vi "test Add and Remove UDP.vi"(8 "error in (no error)":errorcluster, 11 "TestCase in":refnum<class "Add and Remove Test.lvclass">) -> (0 "error out":errorcluster, 3 "TestCase out":refnum<class "Add and Remove Test.lvclass">)   [LabVIEW 2020, in "Add and Remove Test.lvclass"]
uses:
  Add and Remove Test.lvclass
  <vilib>/addons/_JKI Toolkits/VI Tester/TestCase.llb/TestCase.lvclass
  Scripting API/Data Sharing Framework Custom Device Scripting.lvlib
  Includes/DSF Core.lvlibp/Typedefs/DSF Timing Info.ctl
  Includes/DSF Core.lvlibp
  Includes/DSF Core.lvlibp/Typedefs/Core Plugin Configuration.ctl
  Includes/DSF Core.lvlibp/Classes/Configuration/Core/Plugin/Plugin Configuration.lvclass
  Includes/DSF Core.lvlibp/Typedefs/DSF Settings Info.ctl
  Includes/DSF Core.lvlibp/Typedefs/Core Thread Configuration.ctl
  Includes/DSF Core.lvlibp/Classes/Configuration/Core/Thread/Thread Configuration.lvclass
  Includes/DSF Core.lvlibp/Typedefs/DSF Direction.ctl
  Includes/DSF Core.lvlibp/Typedefs/DSF Timeout Behavior.ctl
  Includes/DSF Core.lvlibp/Typedefs/Core Group Configuration.ctl
  Includes/DSF Core.lvlibp/Classes/Configuration/Core/Group/Group Configuration.lvclass
  Includes/DSF Core.lvlibp/Typedefs/Core Transfer Configuration.ctl
  Includes/DSF Core.lvlibp/Classes/Configuration/Core/Transfer/Transfer Configuration.lvclass
  Includes/DSF Core.lvlibp/Typedefs/DSF Data Type.ctl
  Includes/DSF Core.lvlibp/Typedefs/Core Channel Configuration.ctl
  Includes/DSF Core.lvlibp/Classes/Configuration/Core/Channel/Channel Configuration.lvclass
  Includes/DSF Core.lvlibp/Typedefs/DSF Engine Channel Configuration.ctl
  Includes/DSF Core.lvlibp/Typedefs/DSF Engine Transfer Configuration.ctl
  Includes/DSF Core.lvlibp/Typedefs/DSF Engine Transfer Group Configuration.ctl
  Includes/DSF Core.lvlibp/Typedefs/DSF Engine Plugin Thread Configuration.ctl
  Includes/DSF Core.lvlibp/Typedefs/DSF Engine Plugin Configuration.ctl
  Includes/DSF Core.lvlibp/Typedefs/DSF Engine Framework Configuration.ctl
  <vilib>/NI/VeriStand Custom Device Testing Tools/VeriStandTestUtilities/VeriStandTestUtilities.lvlib
  Includes/DSF Core.lvlibp/Classes/Configuration Session/Configuration Session.lvclass
  <vilib>/NI VeriStand/Custom Device API/Custom Device Item Ref.ctl
  <vilib>/NI VeriStand/Custom Device API/Custom Device API.lvlib
  C:/Program Files (x86)/National Instruments/LabVIEW 2020/vi.lib/addons/_JKI Toolkits/VI Tester/TestCase.llb/TestCase.lvclass
  C:/Users/nitest/Desktop/Git/niveristand-data-sharing-framework-custom-device/Source/Custom Device/Tests/Unit/Add and Remove/Add and Remove Test.lvclass
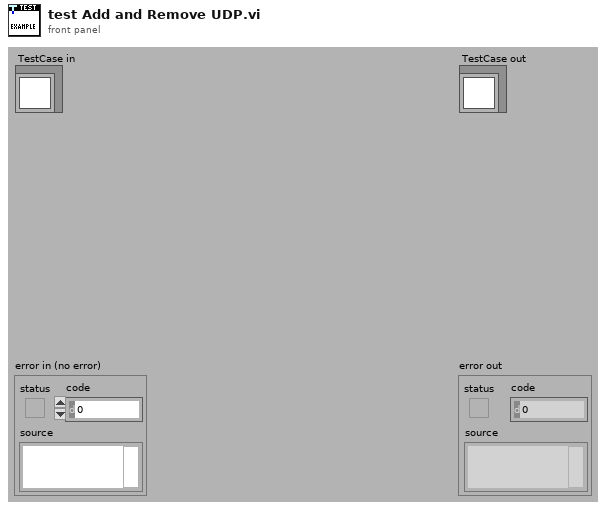
[diagram p1: front panel]
types:
  T1 = typedef "DSF Core.lvlibp/DSF Engine Framework Configuration.ctl" = cluster{"plugins":T2[]}
  T2 = typedef "DSF Core.lvlibp/DSF Engine Plugin Configuration.ctl" = cluster{"core":T3, "component settings":T5[], "threads":T6[]}
  T3 = typedef "DSF Core.lvlibp/Plugin Configuration.lvclass/Core Plugin Configuration.ctl" = cluster{"name":string, "components":string[], "cycle timing":T4}
  T4 = typedef "DSF Core.lvlibp/DSF Timing Info.ctl" = cluster{"priority":u64, "decimation":u64, "offset":u64}
  T5 = typedef "DSF Core.lvlibp/DSF Settings Info.ctl" = cluster{"component":string, "values":cluster{"key":string, "value":string}[]}
  T6 = typedef "DSF Core.lvlibp/DSF Engine Plugin Thread Configuration.ctl" = cluster{"core":T7, "component settings":T5[], "transfer groups":T8[]}
  T7 = typedef "DSF Core.lvlibp/Thread Configuration.lvclass/Core Thread Configuration.ctl" = cluster{"processor":i32, "priority offset":i16}
  T8 = typedef "DSF Core.lvlibp/DSF Engine Transfer Group Configuration.ctl" = cluster{"core":T9, "component settings":T5[], "transfers":T12[]}
  T9 = typedef "DSF Core.lvlibp/Group Configuration.lvclass/Core Group Configuration.ctl" = cluster{"name":string, "direction":T10, "cycle timing":T4, "timeout behavior":T11, "enable conversion":bool}
  T10 = typedef "DSF Core.lvlibp/DSF Direction.ctl" = enum8{"Tx", "Rx"}
  T11 = typedef "DSF Core.lvlibp/DSF Timeout Behavior.ctl" = enum8{"Increment Late Count", "Throw Error"}
  T12 = typedef "DSF Core.lvlibp/DSF Engine Transfer Configuration.ctl" = cluster{"core":T13, "component settings":T5[], "channels":T14[]}
  T13 = typedef "DSF Core.lvlibp/Transfer Configuration.lvclass/Core Transfer Configuration.ctl" = cluster{"name":string}
  T14 = typedef "DSF Core.lvlibp/DSF Engine Channel Configuration.ctl" = cluster{"core":T15, "component settings":T5[]}
  T15 = typedef "DSF Core.lvlibp/Channel Configuration.lvclass/Core Channel Configuration.ctl" = cluster{"name":string, "units":string, "engine data type":T16, "string data type":T16, "string offset":u64}
  T16 = typedef "DSF Core.lvlibp/DSF Data Type.ctl" = enum8{"Bool", "SGL", "DBL", "I8", "I16", "I32", "I64", "U8", "U16", "U32", "U64"}
  T17 = typedef "Custom Device API.lvlib/Custom Device Item Ref.ctl" = u64
  T18 = typedef "DSF Core.lvlibp/DSF Version Info.ctl" = cluster{"major":u32, "minor":u32, "fix":u32, "build":string}
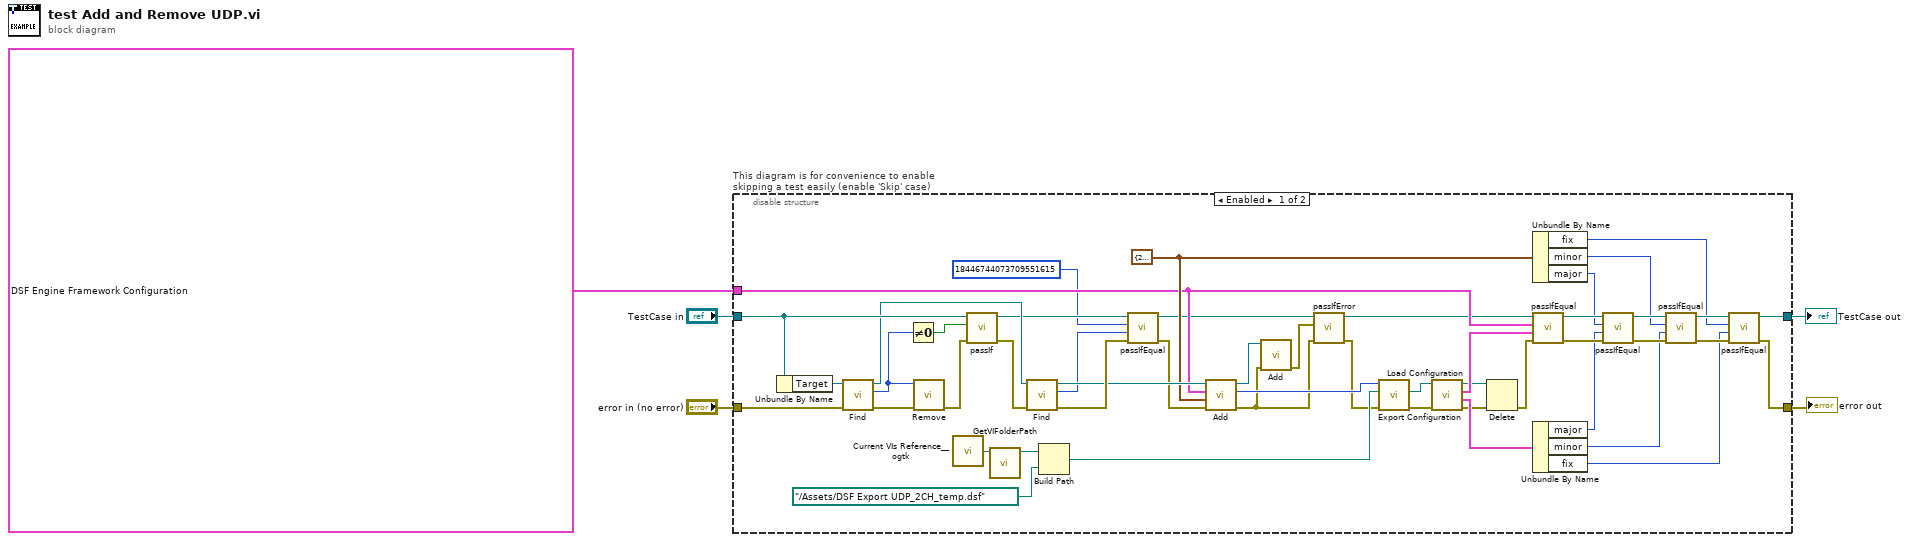
[diagram p0: block diagram]
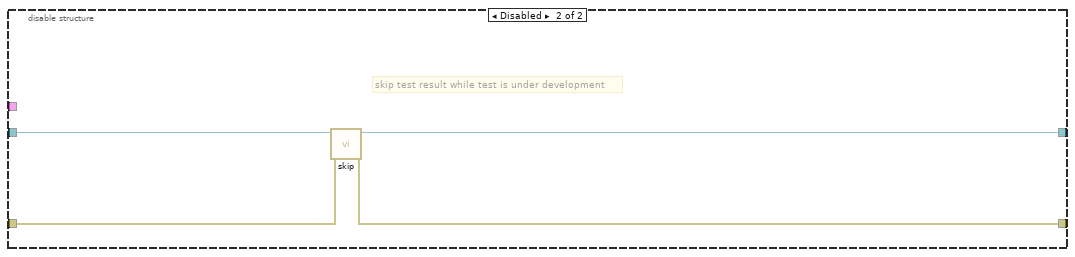
[diagram p2: hidden frame]
diagram:
  n1 = disable-structure "This diagram is for convenience to enable skipping a test easily (enable 'Skip' case)" shown="Enabled" {
    disable-tunnel: "TestCase in" -> [w54 w58]
    disable-tunnel: [w27 w56] -> w2
    disable-tunnel: [w19 w57] -> w4
    disable-tunnel: "error in (no error)" -> [w52 w55]
    disable-tunnel: T1 {"plugins"=[{"core"={"name"="", "components"=["UDP"], "cycle timing"={"priority"=10000, "decimation"=1, "offset"=0}}, "component settings"=[], "threads"=[{"core"={"processor"=-2, "priority offset"=0}, "component settings"=[], "transfer groups"=[{"core"={"name"="Group", "direction"=enum."Tx", "cycle timing"={"priority"=100, "decimation"=1, "offset"=0}, "timeout behavior"=enum."Increment Late Count", "enable conversion"=FALSE}, "component settings"=[], "transfers"=[{"core"={"name"="Transfer"}, "component settings"=[], "channels"=[{"core"={"name"="Voltage", "units"="V", "engine data type"=enum."DBL", "string data type"=enum."DBL", "string offset"=0}, "component settings"=[]}, {"core"={"name"="Current", "units"="A", "engine data type"=enum."DBL", "string data type"=enum."DBL", "string offset"=0}, "component settings"=[]}]}]}]}, {"core"={"processor"=-2, "priority offset"=0}, "component settings"=[], "transfer groups"=[{"core"={"name"="Group", "direction"=enum."Rx", "cycle timing"={"priority"=100, "decimation"=1, "offset"=0}, "timeout behavior"=enum."Increment Late Count", "enable conversion"=FALSE}, "component settings"=[], "transfers"=[{"core"={"name"="Transfer"}, "component settings"=[], "channels"=[{"core"={"name"="Voltage", "units"="V", "engine data type"=enum."DBL", "string data type"=enum."DBL", "string offset"=0}, "component settings"=[]}, {"core"={"name"="Current", "units"="A", "engine data type"=enum."DBL", "string data type"=enum."DBL", "string offset"=0}, "component settings"=[]}]}]}]}]}]} ("framework configuration") -> [w13 _]
    frame Enabled {
      w34 = cluster{"major":u32, "minor":u32, "fix":u32} {"major"=2020, "minor"=3, "fix"=33} ("configuration version")
      n2 = Unbundle By Name(w54) -> ("Target"=w53:refnum<k24>)
      n3 = call "Find.vi"("error in"=w52, "target in"=w53) -> ("error out"=w49:errorcluster, "data sharing framework custom device"=w50:T17, "target out"=w48:refnum<k24>)  [unwired: 6 in, 1 out]
      n4 = Not Equal To 0?(x=w50) -> (x != 0?=w51:bool)
      n5 = call "Remove.vi"("error in"=w49, "data sharing framework custom device"=w50) -> ("error out"=w47:errorcluster)  [unwired: 9 in]
      n6 = call <userlib>:"Current VIs Reference__ogtk.vi"() -> ("Current VI's reference"=w41:refnum<vi>)  [unwired: 5 in]
      n7 = call-dynamic "passIf.vi"("error in (no error)"=w47, "pass"=w51, "TestCase in"=w54) -> ("error out"=w46:errorcluster, "TestCase out"=w45:refnum<class "Add and Remove Test.lvclass">)  [unwired: 7 in]
      n8 = call <vilib>:"GetVIFolderPath.vi"("VI Reference in"=w41) -> ("VI Folder Path out"=w40:path)  [unwired: 9 in, 1 out]
      n9 = call "Find.vi"("error in"=w46, "target in"=w48) -> ("error out"=w44:errorcluster, "data sharing framework custom device"=w8:T17, "target out"=w43:refnum<k24>)  [unwired: 6 in, 1 out]
      n10 = Build Path(base path=w40, name or relative path=path "../Assets/DSF Export UDP_2CH_temp.dsf" ("base path")) -> (appended path=w38:path)
      n11 = call-dynamic "passIfEqual.vi"("error in (no error)"=w44, "y"=w8, "x"=T17 18446744073709551615 ("data sharing framework custom device"), "TestCase in"=w45) -> ("error out"=w42:errorcluster, "TestCase out"=w12:refnum<class "Add and Remove Test.lvclass">)  [unwired: 6 in]
      n12 = call "Add.vi"("error in"=w42, "configuration version"=w34, "framework configuration"=w13, "target in"=w43) -> ("error out"=w9:errorcluster, "data sharing framework custom device"=w15:T17, "target out"=w14:refnum<k24>)  [unwired: 5 in]
      n13 = call "Add.vi"("error in"=w9, "target in"=w14) -> ("error out"=w6:errorcluster)  [unwired: 7 in, 2 out]
      n14 = call-dynamic "passIfError.vi"("error in (no error)"=w9, "error"=w6, "TestCase in"=w12) -> ("error out"=w10:errorcluster, "TestCase out"=w11:refnum<class "Add and Remove Test.lvclass">)  [unwired: 7 in]
      n15 = call "Export Configuration.vi"("error in"=w10, "configuration file path"=w38, "data sharing framework custom device"=w15) -> ("error out"=w36:errorcluster, "actual configuration file path"=w37:path)  [unwired: 6 in, 1 out]
      n16 = call "Load Configuration.vi"("error in (no error)"=w36, "configuration file path"=w37) -> ("error out"=w18:errorcluster, "version"=w35:T18, "framework configuration"=w26:T1, "configuration file path dup"=w16:path)  [unwired: 6 in]
      n17 = Delete(path (use dialog)=w16, error in=w18) -> (error out=w17:errorcluster)  [unwired: 3 in, 2 out]
      n18 = Unbundle By Name(w34) -> ("fix"=w22:u32, "minor"=w20:u32, "major"=w21:u32)
      n19 = call-dynamic "passIfEqual.vi"("error in (no error)"=w17, "y"=w26, "x"=w13, "TestCase in"=w11) -> ("error out"=w32:errorcluster, "TestCase out"=w33:refnum<class "Add and Remove Test.lvclass">)  [unwired: 6 in]
      n20 = Unbundle By Name(w35) -> ("major"=w25:u32, "minor"=w24:u32, "fix"=w23:u32)
      n21 = call-dynamic "passIfEqual.vi"("error in (no error)"=w32, "y"=w25, "x"=w21, "TestCase in"=w33) -> ("error out"=w30:errorcluster, "TestCase out"=w31:refnum<class "Add and Remove Test.lvclass">)  [unwired: 6 in]
      n22 = call-dynamic "passIfEqual.vi"("error in (no error)"=w30, "y"=w24, "x"=w20, "TestCase in"=w31) -> ("error out"=w28:errorcluster, "TestCase out"=w29:refnum<class "Add and Remove Test.lvclass">)  [unwired: 6 in]
      n23 = call-dynamic "passIfEqual.vi"("error in (no error)"=w28, "y"=w23, "x"=w22, "TestCase in"=w29) -> ("error out"=w19:errorcluster, "TestCase out"=w27:refnum<class "Add and Remove Test.lvclass">)  [unwired: 6 in]
    }
    frame Disabled {
      # "skip test result while test is under development"
      n24 = call <vilib>:"skip.vi"("error in (no error)"=w55, "TestCase in"=w58) -> ("error out"=w57:errorcluster, "TestCase out"=w56:refnum<class "Add and Remove Test.lvclass">)  [unwired: 8 in]
    }
  }
  "error out" <- w4
  "TestCase out" <- w2
